vi "校准中 (子VI).vi"(10 "校准按钮":refnum<vi>, 11 "曲线模型":refnum<vi>) -> ()   [LabVIEW 2016]
uses:
  <vilib>/ptbypt/NI_PtbyPt.lvlib
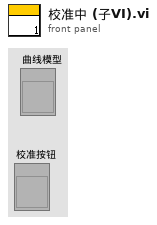
[diagram p1: front panel]
types:
  T1 = enum8{"Enabled", "Disabled", "Disabled and Grayed Out"}
  T2 = cluster{"系统时间":timestamp, "工作状态":u16, "测量模式":enum16{"待机", "连续模式", "周期模式", "定点模式", "受控模式", "手动模式"}, "告警代码":u16, "故障代码":u16, "日志代码":u16, "软件版本":u16, "测量间隔":u16, "消解实时温度":dbl, "校准间隔（天）":u16, "校准间隔（时）":u16, "周期测量时间（23_16）":u16, "周期测量时间（15_0）":u16, "清洗周期（次数）":u16, "运行模式":u16, "自动校准状态":u16, "自动清洗状态":u16}
  T3 = cluster{"公式":cluster{"X^2":dbl, "X":dbl, "B":dbl}, "校准":cluster{"校准？":bool, "校准点1-5":u16, "校准浓度":dbl}}
  T4 = cluster{"标液浓度1":dbl, "测量吸光度1":dbl, "样品1启用":bool, "标液浓度2":dbl, "测量吸光度2":dbl, "样品2启用":bool, "标液浓度3":dbl, "测量吸光度3":dbl, "样品3启用":bool, "标液浓度4":dbl, "测量吸光度4":dbl, "样品4启用":bool, "标液浓度5":dbl, "测量吸光度5":dbl, "样品5启用":bool, "模型":enum32{"线性", "多项式"}, "method":enum16{"最小二乘", "最小绝对残差", "Bisquare"}, "精度":dbl, "XY图":cluster{"X Values":dbl[], "Y Values":dbl[]}[], "拟合公式":string, "r^2":dbl, "零点校准时间":timestamp, "标液校准时间1":timestamp, "标液校准时间2":timestamp, "标液校准时间3":timestamp, "标液校准时间4":timestamp}
  T5 = cluster{"测量量程":dbl, "测量精度":dbl, "测量间隔":dbl, "消解温度":dbl, "消解时长":dbl, "空白校准时间":timestamp, "曲线截距":dbl, "曲线斜率":dbl, "测量检出限":dbl, "测量信号值":dbl, "线性相关系数":dbl, "二次多项式系数":dbl, "标样校准时间":timestamp, "稀释倍数":dbl, "三项式系数":dbl, "空白标定系数":dbl, "量程系数":dbl, "F0/ORPA":dbl, "F1/ORPB":dbl, "F2/ORPK":dbl, "F3":dbl, "F4":dbl, "F5":dbl, "F6":dbl, "F7":dbl, "X0/滴定数":dbl, "量程":dbl}
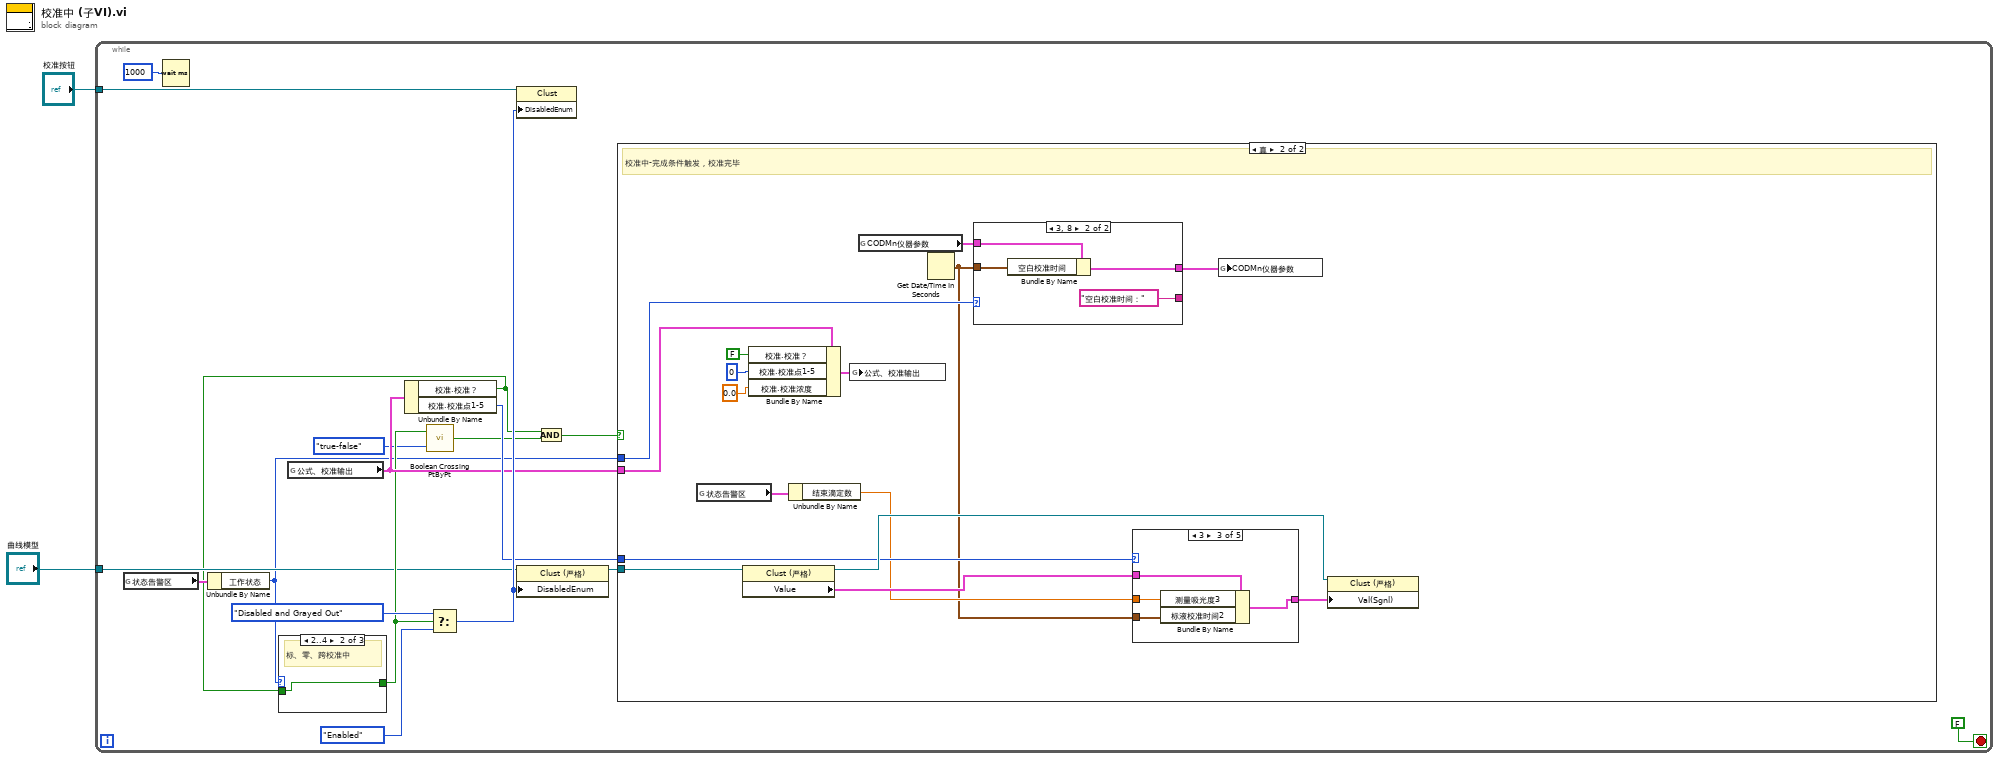
[diagram p0: block diagram]
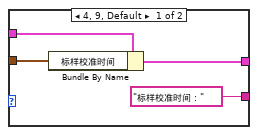
[diagram p3: hidden frame]
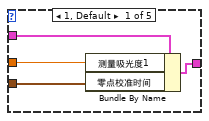
[diagram p4: hidden frame]
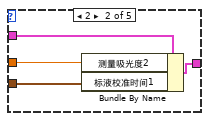
[diagram p5: hidden frame]
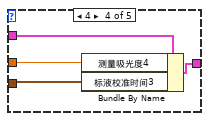
[diagram p6: hidden frame]
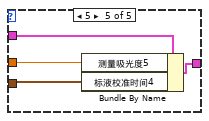
[diagram p7: hidden frame]
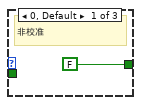
[diagram p8: hidden frame]
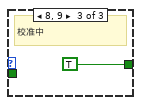
[diagram p9: hidden frame]
diagram:
  n1 = while {
    tunnel: "校准按钮" -> [w6]
    tunnel: "曲线模型" -> [w5]
    stop <- FALSE stop-if-true
    n2 = global read "VAR挥发酚全局变量.vi" "状态告警区"() -> (w19:T2)
    n3 = Wait (ms)(milliseconds to wait=u32 1000 ("等待时间（毫秒）")) -> ()  [unwired: 1 out]
    n4 = Unbundle By Name(w19) -> ("工作状态"=w4:u16)
    n5 = global read "挥发酚断电保存全局变量.vi" "公式、校准输出"() -> (w10:T3)
    n6 = Unbundle By Name(w10) -> ("校准.校准？"=w3:bool, "校准.校准点1-5"=w11:u16)
    n7 = case shown="2..4" w4 {
      tunnel: [FALSE w65 TRUE] -> w9
      tunnel: w3 -> [_ w65 _]
      frame 0, Default {
        # "非校准"
      }
      frame 2..4 {
        # "标、零、跨校准中"
      }
      frame 8, 9 {
        # "校准中"
      }
    }
    n8 = call <vilib>:"Boolean Crossing PtByPt.vi"("direction"=enum16{"either", "false-true", "true-false"}."true-false", "input"=w9) -> ("crossing"=w7:bool)  [unwired: 1 in]
    n9 = Select(t=T1."Disabled and Grayed Out" ("禁用"), s=w9, f=T1."Enabled" ("禁用")) -> (s? t:f=w14:T1)
    n10 = property class="Clust"(reference=w6, "DisabledEnum"=w14) -> ()  [unwired: 1 in, 2 out]
    n11 = property class="Clust (严格)"(reference=w5, "DisabledEnum"=w14) -> (reference out=w12:refnum<vi>)  [unwired: 1 in, 1 out]
    n12 = And(x=w3, y=w7) -> (x .and. y?=w13:bool)
    n13 = case shown="真" w13 {
      tunnel: w12 -> [_ w35]
      tunnel: w11 -> [_ w32]
      tunnel: w10 -> [_ w29]
      tunnel: w4 -> [_ w27]
      frame False {
      }
      frame True {
        # "校准中-完成条件触发，校准完毕"
        n14 = global read "VAR挥发酚全局变量.vi" "状态告警区"() -> (w33:T2)
        n15 = property class="Clust (严格)"(reference=w35) -> (reference out=w34:refnum<vi>, "Value"=w31:T4)  [unwired: 1 in, 1 out]
        n16 = Bundle By Name(cluster=w29, "校准.校准？"=FALSE, "校准.校准点1-5"=u16 0, "校准.校准浓度"=0.0) -> (w21:T3)
        n17 = Unbundle By Name(w33) -> ("结束滴定数"=w28:sgl)
        n18 = global write "挥发酚断电保存全局变量.vi" "公式、校准输出"(w21) -> ()
        n19 = global read "挥发酚断电保存全局变量.vi" "CODMn仪器参数"() -> (w26:T5)
        n20 = Get Date/Time In Seconds() -> (seconds since 1Jan1904=w20:timestamp)
        n21 = case shown="3, 8" w27 {
          tunnel: ["标样校准时间：" "空白校准时间："] -> _
          tunnel: w26 -> [w38 w41]
          tunnel: w20 -> [w37 w42]
          tunnel: [w36 w40] -> w25
          frame 4, 9, Default {
            n22 = Bundle By Name(cluster=w38, "标样校准时间"=w37) -> (w36:T5)
          }
          frame 3, 8 {
            n23 = Bundle By Name(cluster=w41, "空白校准时间"=w42) -> (w40:T5)
          }
        }
        n24 = case shown="3" w32 {
          tunnel: w31 -> [w47 w51 w55 w59 w62]
          tunnel: [w46 w50 w54 w58 w63] -> w30
          tunnel: w28 -> [w45 w49 w53 w57 w61]
          tunnel: w20 -> [w44 w48 w52 w56 w60]
          frame 1, Default {
            n25 = Bundle By Name(cluster=w47, "测量吸光度1"=w45, "零点校准时间"=w44) -> (w46:T4)
          }
          frame 2 {
            n26 = Bundle By Name(cluster=w51, "测量吸光度2"=w49, "标液校准时间1"=w48) -> (w50:T4)
          }
          frame 3 {
            n27 = Bundle By Name(cluster=w55, "测量吸光度3"=w53, "标液校准时间2"=w52) -> (w54:T4)
          }
          frame 4 {
            n28 = Bundle By Name(cluster=w59, "测量吸光度4"=w57, "标液校准时间3"=w56) -> (w58:T4)
          }
          frame 5 {
            n29 = Bundle By Name(cluster=w62, "测量吸光度5"=w61, "标液校准时间4"=w60) -> (w63:T4)
          }
        }
        n30 = global write "挥发酚断电保存全局变量.vi" "CODMn仪器参数"(w25) -> ()
        n31 = property class="Clust (严格)"(reference=w34, "Val(Sgnl)"=w30) -> ()  [unwired: 1 in, 2 out]
      }
    }
  }
